vi "Init.vi"(8 "error in (no error)":errorcluster, 10 "Instrument String":variant, 11 "NI DMM in":refnum<class "NI DMM.lvclass">) -> (0 "error out":errorcluster, 2 "Found?":bool=TRUE, 3 "NI DMM out":refnum<class "NI DMM.lvclass">)   [LabVIEW 2025, in "DMM.lvlib" / "NI DMM.lvclass"]
uses:
  NI DMM.lvclass
  DMM configuration/DMM configuration.lvclass
  NI DMM.lvclass/NI DMM.ctl
  Users/Public/Documents/Sandia National Labs/TSS Plugin/Abstract Engine.lvlibp/Plugin/Abstract/Instrument configuration/Read Instrument Setting.vi
  Users/Public/Documents/Sandia National Labs/TSS Plugin/CEF.lvlibp/serializable configuration/CEF_serializable configuration.lvclass
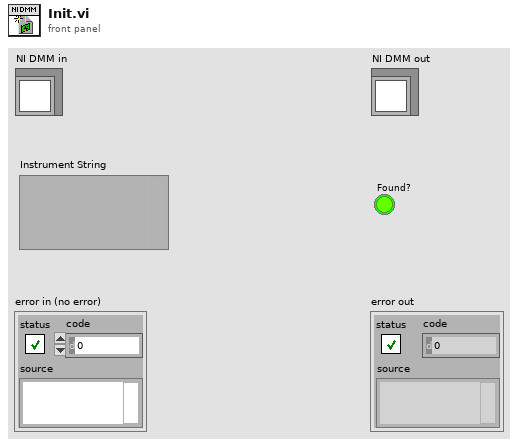
[diagram p1: front panel]
types:
  T1 = typedef "Abstract Engine.lvlibp/Instrument configuration.lvclass/Default Instrument.ctl" = cluster{"Type":string, "Address":string, "SW Alias":string, "Description":string, "Enabled":bool}
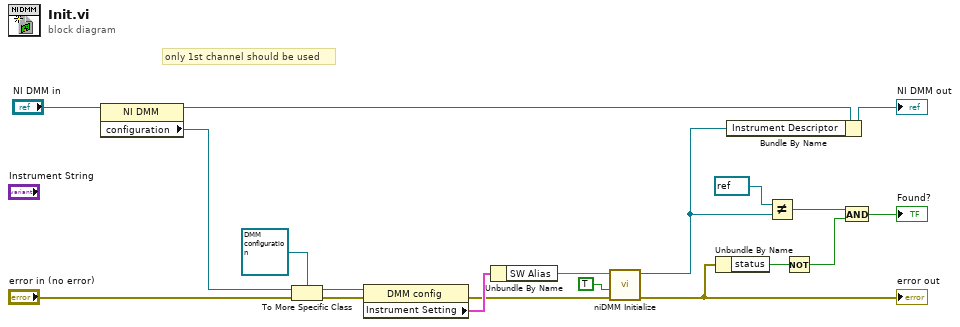
[diagram p0: block diagram]
diagram:
  # "only 1st channel should be used"
  n1 = property class="NI DMM"(reference="NI DMM in") -> (reference out=w1:refnum<class "NI DMM.lvclass">, "configuration"=w12:refnum<class "CEF_serializable configuration.lvclass">)  [unwired: 1 in, 1 out]
  n2 = To More Specific Class(target class=refnum<class "DMM configuration.lvclass"> refnum ("DMM.lvlib:DMM configuration.lvclass"), reference=w12, error in="error in (no error)") -> (specific class reference=w13:refnum<class "DMM configuration.lvclass">, error out=w10:errorcluster)
  n3 = property class="DMM config"(reference=w13, error in=w10) -> (error out=w2:errorcluster, "Instrument Setting"=w3:T1)  [unwired: 1 out]
  n4 = Unbundle By Name(w3) -> ("SW Alias"=w14:string)
  n5 = call <instrlib>:"niDMM Initialize.vi"("error in (no error)"=w2, "Reset"=TRUE, "Instrument Descriptor"=w14) -> ("error out"=w7:errorcluster, "instrument handle out"=w17:refnum<k15>)  [unwired: 7 in]
  "error out" <- w7
  n6 = Unbundle By Name(w7) -> ("status"=w8:bool)
  n7 = Bundle By Name(cluster=w1, "Instrument Descriptor"=w17) -> (→"NI DMM out":refnum<class "NI DMM.lvclass">)
  n8 = Not Equal?(x=refnum<k15> refnum ("instrument handle out"), y=w17) -> (x != y?=w6:bool)
  n9 = Not(x=w8) -> (.not. x?=w5:bool)
  n10 = And(x=w6, y=w5) -> (x .and. y?=→"Found?":bool)
